vi "Start Sync.vi"(8 "error in (no error)":errorcluster, 11 "gRPC Server in":refnum<class "Communicate.lvclass">) -> (0 "error out":errorcluster, 3 "gRPC Server out":refnum<class "Communicate.lvclass">)   [LabVIEW 2021, in "Demo_server.lvlib" / "Communicate.lvclass"]
uses:
  Communicate.lvclass
  Communicate.lvclass/Communicate.ctl
  RPC Messages/Communication_ActionReply.ctl
  Demo_server.lvlib
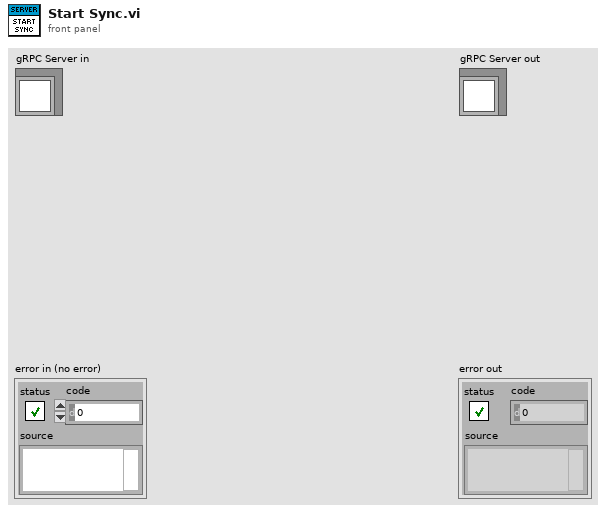
[diagram p1: front panel]
types:
  T1 = typedef "Demo_server.lvlib/Communication_ActionReply.ctl" = cluster{"Reply":string, "Status":string}
  T2 = typedef "Demo_server.lvlib/Communicate.lvclass/Server Internal UEs.ctl" = cluster{"Communicate Transmission Internal UE":refnum<user-event>}
  T3 = typedef "Demo_server.lvlib/Communicate.lvclass/Server gRPC UEs.ctl" = cluster{"Communicate Transmission gRPC UE":refnum<user-event>}
  T4 = typedef "grpc-lvsupport-release.lvlib/grpcId.ctl" = u64
  T5 = typedef "Demo_server.lvlib/Communication_ActionRequest.ctl" = cluster{"Request":string, "Data":string}
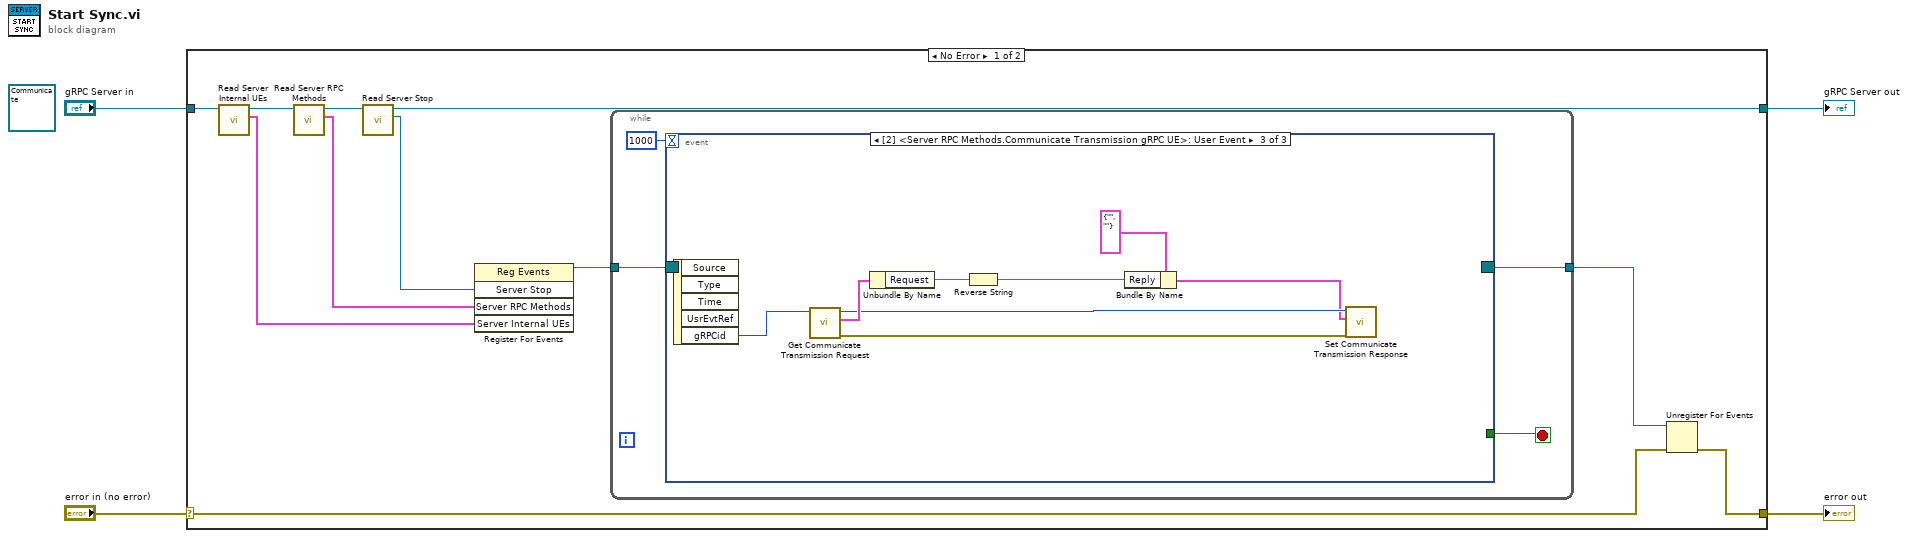
[diagram p0: block diagram]
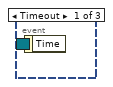
[diagram p2: hidden frame]
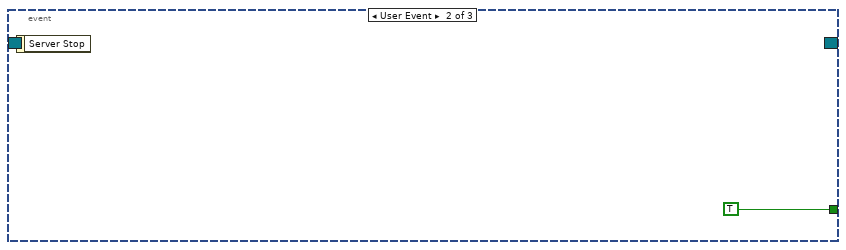
[diagram p3: hidden frame]
diagram:
  (unwired) refnum<class "Communicate.lvclass"> refnum ("gRPC Server in")
  n1 = case shown="No Error" "error in (no error)" {
    selector: "error in (no error)" -> [w9 w30]
    tunnel: [w8 w30] -> w3
    tunnel: [w5 w29] -> w1
    tunnel: "gRPC Server in" -> [w15 w29]
    frame No Error {
      n2 = call "Read Server Internal UEs.vi"("SignalGeneratorService in"=w15) -> ("Server Internal UEs"=w13:T2, "SignalGeneratorService out"=w14:refnum<class "Communicate.lvclass">)  [unwired: 8 in, 1 out]
      n3 = call "Read Server RPC Methods.vi"("SignalGeneratorService in"=w14) -> ("Server RPC Methods"=w7:T3, "SignalGeneratorService out"=w12:refnum<class "Communicate.lvclass">)  [unwired: 8 in, 1 out]
      n4 = call-dynamic "Read Server Stop.vi"("iService in"=w12) -> ("Server Stop"=w6:refnum<user-event>, "iService out"=w5:refnum<class "Communicate.lvclass">)  [unwired: 8 in, 1 out]
      n5 = register-events(w6, w7, w13) -> (reference out=w11:refnum<event-registration>)  [unwired: 2 in, 1 out]
      n6 = while {
        tunnel: w11 -> [w19]
        tunnel: [w17] -> w10
        stop <- w18 stop-if-true
        n7 = event "RPC Methods Event Structure" shown="[2] <Server RPC Methods.Communicate Transmission gRPC UE>: User Event" {
          selector: w19 -> [_ _ _]
          dyn-events: [_ _ _] -> w17
          timeout: 1000 -> [_ _ _]
          tunnel: [_ TRUE _] -> w18
          event Timeout {
            n8 = event-data() -> ()  [unwired: 1 in, 1 out]
          }
          event User Event {
            n9 = event-data() -> ()  [unwired: 1 in, 1 out]
          }
          event User Event {
            n10 = event-data() -> ("gRPCid"=w21:T4)  [unwired: 1 in, 4 out]
            n11 = call "Get Communicate Transmission Request.vi"("gRPCid in"=w21) -> ("error out"=w25:errorcluster, "Message Data"=w26:T5, "gRPCid out"=w24:T4)  [unwired: 8 in]
            n12 = Unbundle By Name(w26) -> ("Request"=w27:string)
            n13 = Reverse String(1:w27) -> (0:w28:string)
            n14 = Bundle By Name(cluster=T1 {"Reply"="", "Status"=""} ("Message Data"), "Reply"=w28) -> (w22:T1)
            n15 = call "Set Communicate Transmission Response.vi"("error in (no error)"=w25, "Message Data"=w22, "gRPCid in"=w24) -> ()  [unwired: 8 in, 1 out]
          }
        }
      }
      n16 = Unregister For Events(event registration refnum=w10, error in=w9) -> (error out=w8:errorcluster)
    }
    frame Error {
    }
  }
  "error out" <- w3
  "gRPC Server out" <- w1
